vi "ErrorLog_ShowErrorDialog.vi"(8 "error in (no error)":errorcluster, 11 "reference in":refnum<class "ErrorLog.lvclass">) -> (0 "error out":errorcluster, 3 "reference out":refnum<class "ErrorLog.lvclass">)   [LabVIEW 2014, in "ErrorLog.lvclass"]
doc: "Shows Error Dialog"
uses:
  ErrorLog.lvclass
panel:
  in  "pop":bool
  in  "CLR":bool
  out "Errors":string
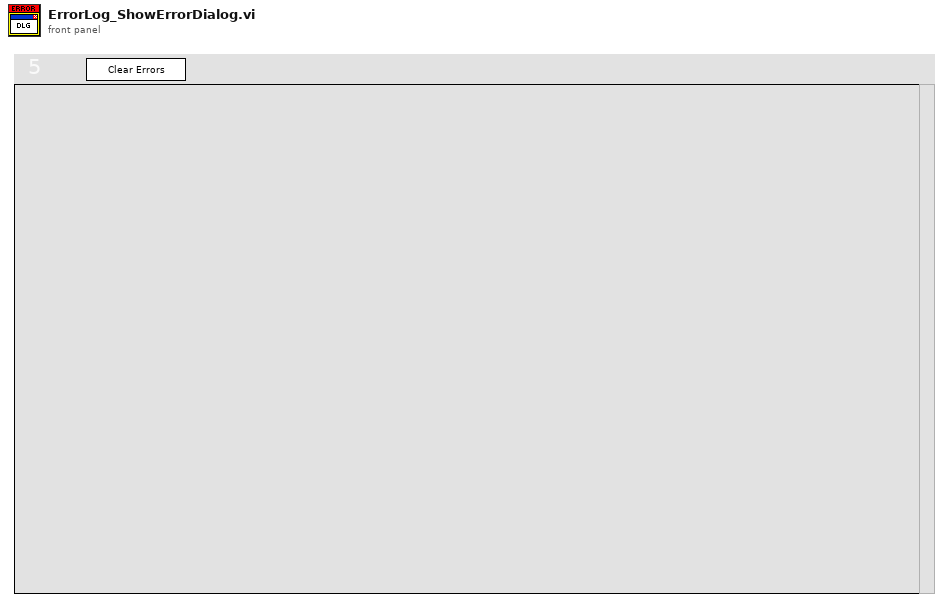
[diagram p1: front panel]
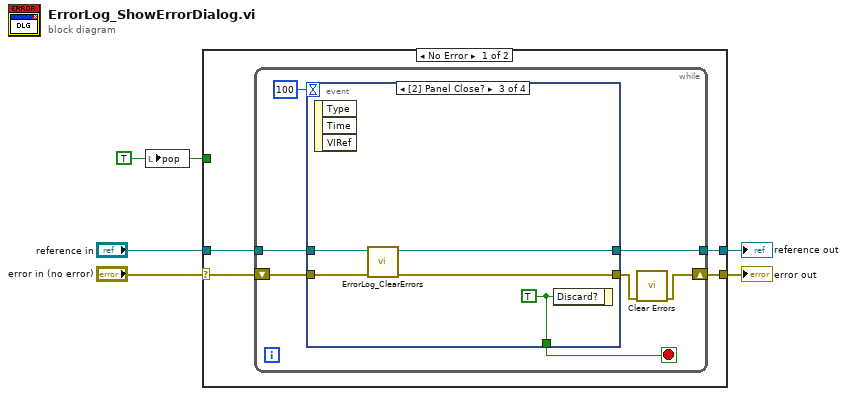
[diagram p0: block diagram]
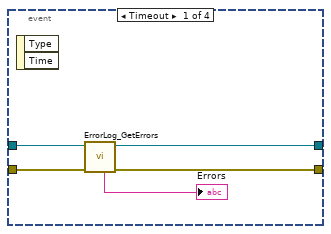
[diagram p2: hidden frame]
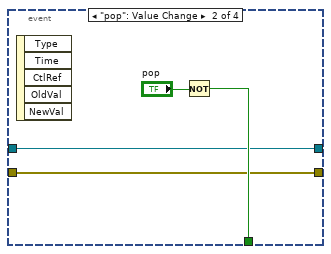
[diagram p3: hidden frame]
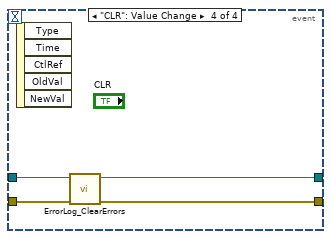
[diagram p4: hidden frame]
diagram:
  w3 = TRUE
  n1 = local write "pop"(w3) -> ()
  n2 = case shown="No Error" "error in (no error)" {
    selector: "error in (no error)" -> [w8 w35]
    tunnel: "reference in" -> [w9 w36]
    tunnel: w3 -> [_ _]
    tunnel: [w7 w36] -> w2
    tunnel: [w6 w35] -> w1
    frame No Error {
      n3 = while {
        shift-right: [w11] -> w6
        shift-left: w8 -> [w15]
        tunnel: w9 -> [w13]
        tunnel: [w12] -> w7
        stop <- w14 stop-if-true
        n4 = event shown="[2] Panel Close?" {
          selector: _ -> [_ _ _ _]
          dyn-events: _ -> [_ _ _ _]
          timeout: 100 -> [_ _ _ _]
          tunnel: w15 -> [w21 w23 w28 w33]
          tunnel: [w19 w23 w26 w31] -> w10
          tunnel: [_ w24 w30 _] -> w14
          tunnel: w13 -> [w18 w22 w29 w34]
          tunnel: [w17 w22 w27 w32] -> w12
          event Timeout {
            n5 = event-data() -> ()  [unwired: 1 in, 2 out]
            n6 = call-dynamic "ErrorLog_GetErrors.vi"("error in (no error)"=w21, "reference in"=w18) -> ("error out"=w19:errorcluster, "reference out"=w17:refnum<class "ErrorLog.lvclass">, "Errors since last clear"=→"Errors":string)  [unwired: 4 in, 3 out]
          }
          event "pop": Value Change {
            n7 = event-data() -> ()  [unwired: 1 in, 5 out]
            n8 = Not(x="pop") -> (.not. x?=w24:bool)
          }
          event Panel Close? {
            w30 = TRUE ("Discard?")
            n9 = event-data() -> ()  [unwired: 1 in, 3 out]
            n10 = call-dynamic "ErrorLog_ClearErrors.vi"("error in (no error)"=w28, "reference in"=w29) -> ("error out"=w26:errorcluster, "reference out"=w27:refnum<class "ErrorLog.lvclass">)  [unwired: 8 in]
            n11 = event-data("Discard?"=w30) -> ()  [unwired: 1 in, 1 out]
          }
          event "CLR": Value Change {
            n12 = event-data() -> ()  [unwired: 1 in, 5 out]
            n13 = call-dynamic "ErrorLog_ClearErrors.vi"("error in (no error)"=w33, "reference in"=w34) -> ("error out"=w31:errorcluster, "reference out"=w32:refnum<class "ErrorLog.lvclass">)  [unwired: 8 in]
          }
        }
        n14 = call <vilib>:"Clear Errors.vi"("error in (no error)"=w10) -> ("error out"=w11:errorcluster)  [unwired: 5 in, 1 out]
      }
    }
    frame Error {
    }
  }
  "error out" <- w1
  "reference out" <- w2
